vi "Create Default Attributes.vi"(5 "Unique ID":string, 7 "Process Executive Ref":refnum<data-value>, 11 "Start Tire Shine Foam in":refnum<class "Start Tire Shine Foam.lvclass">) -> (3 "Start Tire Shine Foam out":refnum<class "Start Tire Shine Foam.lvclass">)   [LabVIEW 2019, in "Start Tire Shine Foam.lvclass"]
uses:
  <vilib>/gpm_packages/@cs/Car-wash/Source/Process Steps/Start Tire Shine Foam/Start Tire Shine Foam.lvclass
  <vilib>/gpm_packages/@cs/test-executive/Source/Test Executive/ITestExecutive/ITest Executive.lvclass
  293ec867-f382-4e6d-a471-dccc023b648a.vi
  <vilib>/Utility/error.llb/Error Cluster From Error Code.vi
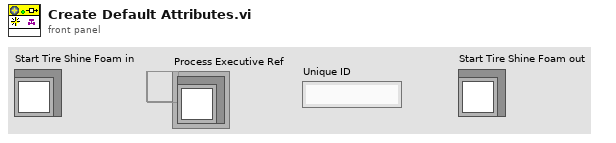
[diagram p1: front panel]
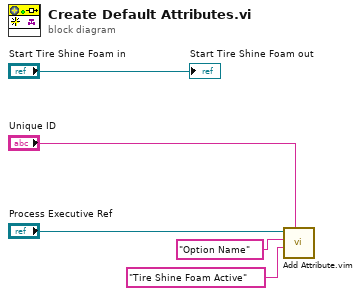
[diagram p0: block diagram]
diagram:
  n1 = call "Add Attribute.vim"("ID"="Unique ID", "Attribute"="Tire Shine Foam Active" ("Item Name"), "Attribute Name"="Option Name" ("Item Name"), "Test Executive Ref"="Process Executive Ref") -> ()  [unwired: 4 in, 4 out]
  "Start Tire Shine Foam out" <- "Start Tire Shine Foam in"
